vi "Update Parent and Children Links.vi"(11 "Item Graph In":T1[](array[typedef])) -> (3 "Item Graph":T1[](array[typedef]))   [LabVIEW 2020, in "TypeGraph.lvlib"]
uses:
  TypeGraph.lvlib
  Type Reflection Item.ctl
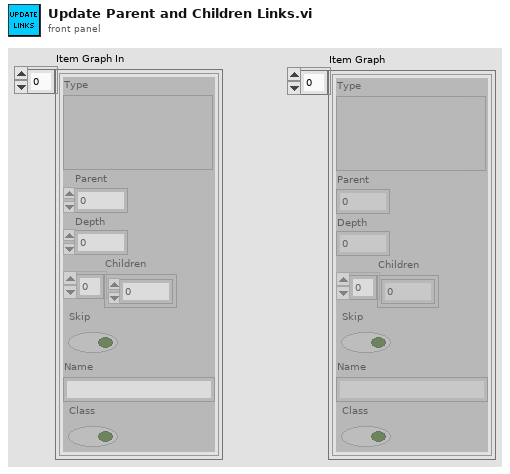
[diagram p1: front panel]
types:
  T1 = typedef "TypeGraph.lvlib/Type Reflection Item.ctl" = cluster{"Type":variant, "Parent":i32, "Depth":i32, "Children":i32[], "Skip":bool, "Name":string, "Class":bool}
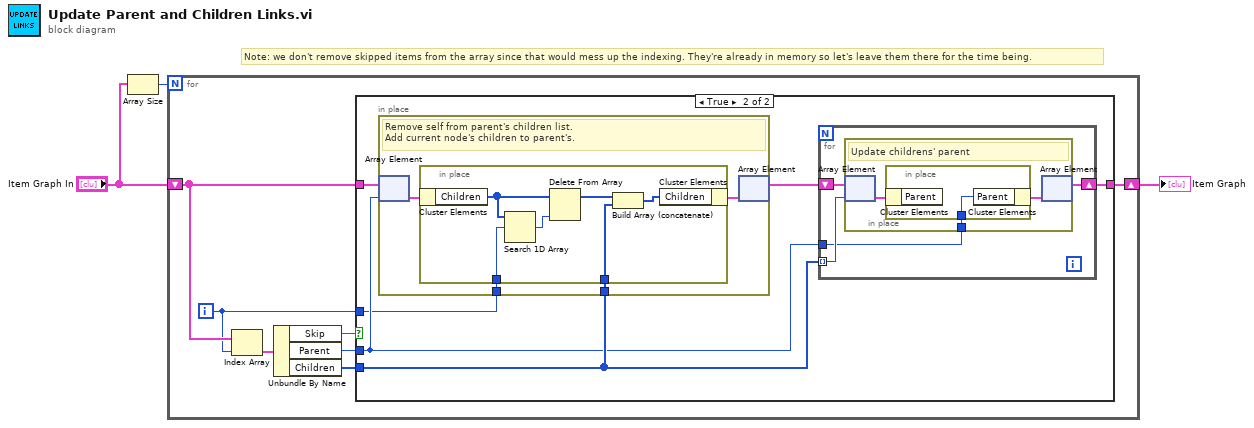
[diagram p0: block diagram]
diagram:
  # "Note: we don't remove skipped items from the array since that would mess up the indexing. They're already in memory so let's leave them there for the time being."
  n1 = Array Size(array="Item Graph In") -> (size(s)=w2:i32)
  n2 = for {
    N: w2 -> [_]
    shift-right: [w7] -> w3
    shift-left: "Item Graph In" -> [w8]
    i -> [w4]
    n3 = Index Array(array=w8, index=w4) -> (element=w10:T1)
    n4 = Unbundle By Name(w10) -> ("Skip"=w9:bool, "Parent"=w6:i32, "Children"=w5:i32[])
    n5 = case shown="True" w9 {
      tunnel: w8 -> [w11 w17]
      tunnel: [w11 w13] -> w7
      tunnel: w6 -> [_ w14]
      tunnel: w5 -> [_ w15]
      tunnel: w4 -> [_ w12]
      frame False {
      }
      frame True {
        n6 = in-place {
          in-place-border: w15 -> [w28]
          in-place-border: w12 -> [w26]
          # "Remove self from parent's children list.\nAdd current node's children to parent's."
          n7 = in-place-array #1(w17, w14) -> (w29:T1)
          n8 = in-place {
            in-place-border: w28 -> [w35]
            in-place-border: w26 -> [w30]
            n9 = in-place-cluster #2(w29) -> ("Children"=w33:i32[])
            n10 = Search 1D Array(1D array=w33, element=w30) -> (index of element=w31:i32)  [unwired: 1 in]
            n11 = Delete From Array(array=w33, index=w31) -> (array with subset deleted=w32:i32[])  [unwired: 1 in, 1 out]
            n12 = Build Array (concatenate)(w32, w35) -> (w34:i32[])
            n13 = in-place-cluster #2("Children"=w34) -> (w27:T1)
          }
          n14 = in-place-array #1(w27) -> (w16:T1[])  [unwired: 1 out]
        }
        n15 = for {
          shift-right: [w18] -> w13
          shift-left: w16 -> [w21]
          tunnel: w15 -> [w20] mode=indexing
          tunnel: w14 -> [w19]
          n16 = in-place {
            in-place-border: w19 -> [w23]
            # "Update childrens' parent"
            n17 = in-place-array #3(w21, w20) -> (w24:T1)
            n18 = in-place {
              in-place-border: w23 -> [w25]
              n19 = in-place-cluster #4(w24) -> ()  [unwired: 1 out]
              n20 = in-place-cluster #4("Parent"=w25) -> (w22:T1)
            }
            n21 = in-place-array #3(w22) -> (w18:T1[])  [unwired: 1 out]
          }
        }
      }
    }
  }
  "Item Graph" <- w3
